vi "Release 1.vi"() -> ()   [LabVIEW 2020, in "Acquisition.lvlib"]
uses:
  Acquisition.lvlib
panel:
  out "Waveform Graph":dbl[](graph)
  in  "Cancel":bool
  in  "Stop":bool
  in  "Start":bool
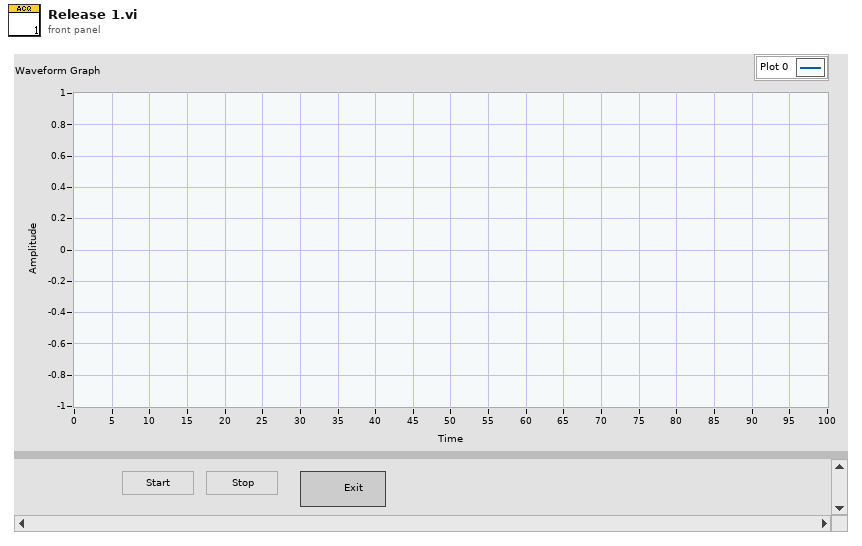
[diagram p1: front panel]
types:
  T1 = typedef "Acquisition.lvlib/Broadcast Events--cluster.ctl" = cluster{"Module Did Init":refnum<user-event>, "Status Updated":refnum<user-event>, "Error Reported":refnum<user-event>, "Module Did Stop":refnum<user-event>, "Update Module Execution Status":refnum<user-event>, "Data Acquired":refnum<user-event>}
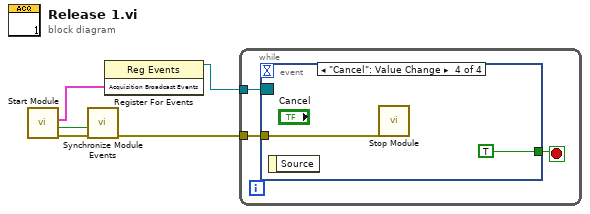
[diagram p0: block diagram]
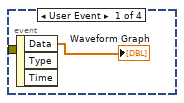
[diagram p2: hidden frame]
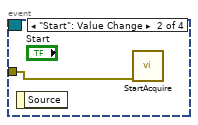
[diagram p3: hidden frame]
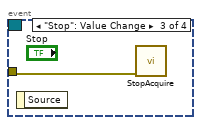
[diagram p4: hidden frame]
diagram:
  n1 = call "Start Module.vi"() -> ("error out"=w3:errorcluster, "Wait for Event Sync?"=w1:bool, "Acquisition Broadcast Events"=w5:T1)  [unwired: 8 in, 1 out]
  n2 = call "Synchronize Module Events.vi"("error in (no error)"=w3, "Wait for Event Sync?"=w1) -> ("error out"=w2:errorcluster)  [unwired: 9 in]
  n3 = register-events(w5) -> (reference out=w4:refnum<event-registration>)  [unwired: 2 in, 1 out]
  n4 = while {
    tunnel: w4 -> [w8]
    tunnel: w2 -> [w7]
    stop <- w6 stop-if-true
    n5 = event shown="[3] \"Cancel\": Value Change" {
      selector: w8 -> [_ _ _ _]
      dyn-events: _ -> [_ _ _ _]
      timeout: _ -> [_ _ _ _]
      tunnel: w7 -> [_ w10 w11 w13]
      tunnel: [_ _ _ TRUE] -> w6
      event User Event {
        n6 = event-data() -> ("Data"=→"Waveform Graph":dbl[])  [unwired: 1 in, 2 out]
      }
      event "Start": Value Change {
        n7 = event-data() -> ()  [unwired: 1 in, 1 out]
        n8 = call "StartAcquire.vi"("error in (no error)"=w10) -> ()  [unwired: 10 in, 1 out]
      }
      event "Stop": Value Change {
        n9 = event-data() -> ()  [unwired: 1 in, 1 out]
        n10 = call "StopAcquire.vi"("error in (no error)"=w11) -> ()  [unwired: 10 in, 1 out]
      }
      event "Cancel": Value Change {
        n11 = event-data() -> ()  [unwired: 1 in, 1 out]
        n12 = call "Stop Module.vi"("error in (no error)"=w13) -> ()  [unwired: 10 in, 1 out]
      }
    }
  }
